vi "Show Hide Tab VIs.vi"(8 "error in (no error)":errorcluster, 10 "Front Panel State":T1(ring), 11 "Panel Names":string[](array[string])) -> (0 "error out":errorcluster)   [LabVIEW 2011]
uses:
  Panel Global Methods.ctl
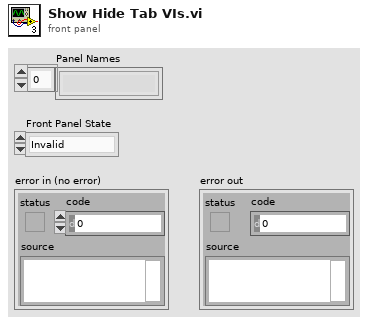
[diagram p1: front panel]
types:
  T1 = enum32{"Invalid", "Standard", "Closed", "Hidden", "Minimized", "Maximized"}
  T2 = typedef "Panel Global Methods.ctl" = enum16{"Read All Panels", "Read Panel Data", "Write Panel Data"}
  T3 = typedef "Panel Data.ctl" = cluster{"Panel VI Name":string, "Hwnd":u32, "Collapsed?":bool, "Panel Ref":refnum<vi>, "Events Variant":variant, "Resizeable?":bool, "Un-Dockedable?":bool, "Docked?":bool}
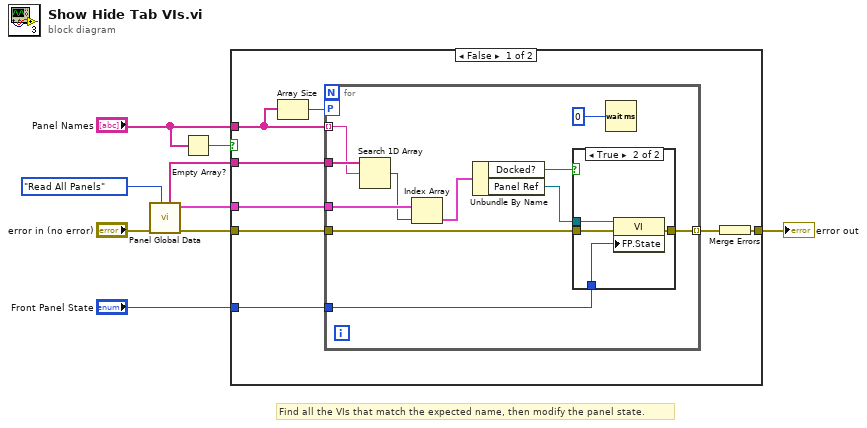
[diagram p0: block diagram]
diagram:
  # "Find all the VIs that match the expected name, then modify the panel state."
  n1 = call "Panel Global Data.vi"("Method (Read All)"=Panel_Global_Methods."Read All Panels", "error in (no error)"="error in (no error)") -> ("error out"=w7:errorcluster, "All Panel Data"=w5:T3[], "Panel VI Names"=w4:string[])  [unwired: 6 in, 1 out]
  n2 = Empty Array?(array="Panel Names") -> (empty?=w1:bool)
  n3 = case shown="False" w1 {
    tunnel: "Panel Names" -> [w16 _]
    tunnel: [w15 w34] -> w9
    tunnel: w7 -> [w13 w34]
    tunnel: "Front Panel State" -> [w12 _]
    tunnel: w5 -> [w11 _]
    tunnel: w4 -> [w10 _]
    frame False {
      n4 = Array Size(array=w16) -> (size(s)=w17:i32)
      n5 = for {
        tunnel: w10 -> [w28]
        tunnel: w11 -> [w26]
        tunnel: w16 -> [w27] mode=indexing
        tunnel: w12 -> [w22]
        tunnel: [w21] -> w14 mode=indexing
        tunnel: w13 -> [w20]
        workers-P: w17 -> [_]
        n6 = Search 1D Array(1D array=w28, element=w27) -> (index of element=w25:i32)  [unwired: 1 in]
        n7 = Index Array(array=w26, index=w25) -> (element=w24:T3)
        n8 = Unbundle By Name(w24) -> ("Docked?"=w18:bool, "Panel Ref"=w23:refnum<vi>)
        n9 = case shown="True" w18 {
          tunnel: w23 -> [_ w33]
          tunnel: w22 -> [_ w32]
          tunnel: [w29 w31] -> w21
          tunnel: w20 -> [w29 w30]
          frame False {
          }
          frame True {
            n10 = property class="VI"(reference=w33, error in=w30, "FP.State"=w32) -> (error out=w31:errorcluster)  [unwired: 1 out]
          }
        }
        n11 = Wait (ms)(milliseconds to wait=u32 0) -> ()  [unwired: 1 out]
      }
      n12 = Merge Errors(w14) -> (w15:errorcluster)
    }
    frame True {
    }
  }
  "error out" <- w9
